vi "FGV read params.vi"(7 "Write (F)":bool, 11 "params in":string) -> (3 "params out":string)   [LabVIEW 2021, in "STAV lib.lvlib"]
uses:
  STAV lib.lvlib
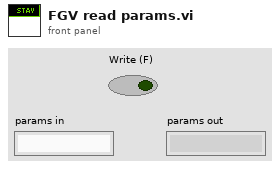
[diagram p1: front panel]
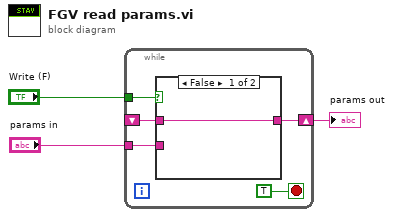
[diagram p0: block diagram]
diagram:
  n1 = while {
    tunnel: "params in" -> [w5]
    tunnel: "Write (F)" -> [w7]
    shift-right: [w6] -> w1
    shift-left: _ -> [w4]
    stop <- TRUE stop-if-true
    n2 = case shown="False" w7 {
      tunnel: [w9 w10] -> w6
      tunnel: w5 -> [_ w10]
      tunnel: w4 -> [w9 _]
      frame False {
      }
      frame True {
      }
    }
  }
  "params out" <- w1
